vi "边写边读文件.vi"() -> ()   [LabVIEW 2017]
panel:
  out "副本文件名":string
  in  "读取后删除副本":bool
  out "读取内容":string
  in  "读取":bool
  in  "停止":bool
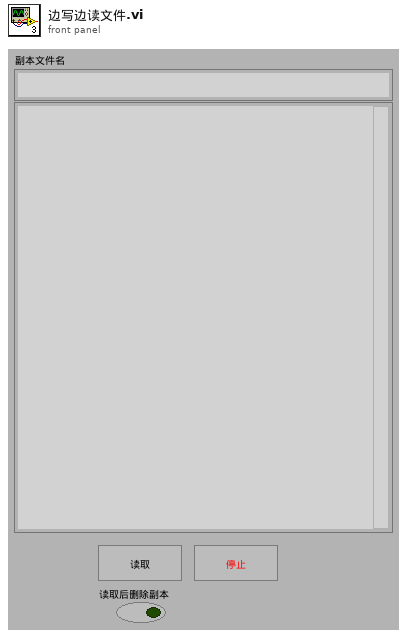
[diagram p1: front panel]
types:
  T1 = enum16{"open", "replace", "create", "open or create", "replace or create", "replace or create with confirmation"}
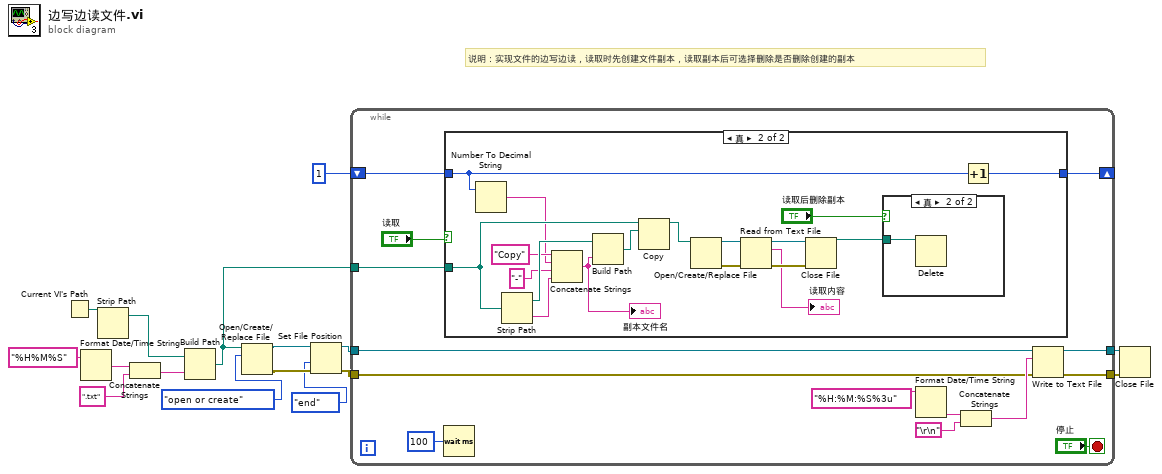
[diagram p0: block diagram]
diagram:
  # "说明：实现文件的边写边读，读取时先创建文件副本，读取副本后可选择删除是否删除创建的副本"
  n1 = Current VI's Path() -> (path=w9:path)
  n2 = Format Date/Time String(time format string (%c)="%H%M%S" ("时间格式字符串(%c)")) -> (date/time string=w13:string)  [unwired: 2 in]
  n3 = Strip Path(path=w9) -> (stripped path=w14:path)  [unwired: 1 out]
  n4 = Concatenate Strings(w13, ".txt" ("字符串")) -> (w12:string)
  n5 = Build Path(base path=w14, name or relative path=w12) -> (appended path=w2:path)
  n6 = Open/Create/Replace File(file path (use dialog)=w2, operation (0:open)=T1."open or create" ("操作(0:open)")) -> (refnum out=w11:refnum<file>, error out=w10:errorcluster)  [unwired: 4 in, 1 out]
  n7 = Set File Position(refnum=w11, from (0:start)=enum16{"start", "end", "current"}."end" ("自（0:起始）"), error in=w10) -> (refnum out=w3:refnum<file>, error out=w4:errorcluster)  [unwired: 1 in]
  n8 = while {
    tunnel: [w26] -> w16
    tunnel: [w25] -> w15
    tunnel: w4 -> [w23]
    tunnel: w3 -> [w22]
    tunnel: w2 -> [w20]
    shift-right: [w17] -> _
    shift-left: 1 -> [w18]
    stop <- "停止" stop-if-true
    n9 = Wait (ms)(milliseconds to wait=u32 100 ("等待时间（毫秒）")) -> ()  [unwired: 1 out]
    n10 = case shown="真" "读取" {
      tunnel: w20 -> [_ w49]
      tunnel: w18 -> [w31 w37]
      tunnel: [w31 w38] -> w17
      frame False {
      }
      frame True {
        n11 = Number To Decimal String(number=w37) -> (decimal integer string=w35:string)  [unwired: 1 in]
        n12 = Strip Path(path=w49) -> (stripped path=w48:path, name=w33:string)
        n13 = Concatenate Strings("Copy" ("字符串"), w35, "-" ("字符串"), w33) -> (w32:string)
        "副本文件名" <- w32
        n14 = Build Path(base path=w48, name or relative path=w32) -> (appended path=w47:path)
        n15 = Copy(10:w47, 11:w49) -> (3:w46:path)  [unwired: 3 in, 2 out]
        n16 = Open/Create/Replace File(file path (use dialog)=w46) -> (refnum out=w45:refnum<file>, error out=w44:errorcluster)  [unwired: 5 in, 1 out]
        n17 = Read from Text File(file (use dialog)=w45, error in=w44) -> (refnum out=w43:refnum<file>, text=→"读取内容":string, error out=w42:errorcluster)  [unwired: 2 in, 1 out]
        n18 = Close File(refnum=w43, error in=w42) -> (path=w40:path)  [unwired: 1 out]
        n19 = case shown="真" "读取后删除副本" {
          tunnel: w40 -> [_ w50]
          frame False {
          }
          frame True {
            n20 = Delete(path (use dialog)=w50) -> ()  [unwired: 4 in, 3 out]
          }
        }
        n21 = Increment(x=w37) -> (x+1=w38:i32)
      }
    }
    n22 = Format Date/Time String(time format string (%c)="%H:%M:%S%3u" ("时间格式字符串(%c)")) -> (date/time string=w28:string)  [unwired: 2 in]
    n23 = Concatenate Strings(w28, "\r\n") -> (w27:string)
    n24 = Write to Text File(file (use dialog)=w22, text=w27, error in=w23) -> (refnum out=w26:refnum<file>, error out=w25:errorcluster)  [unwired: 1 in, 1 out]
  }
  n25 = Close File(refnum=w16, error in=w15) -> ()  [unwired: 2 out]
